vi "Unregister All.vi"() -> (3 "loggers":refnum<class "Logger.lvclass">[](array[class]))   [LabVIEW 2018, in "Logging.lvlib" / "Registry.lvlib"]
uses:
  Registry.lvlib
  Logger/Logger.lvclass
  Registry Actions.ctl
  Utilities/Utilities.lvlib
panel:
  # "Connector Pane"
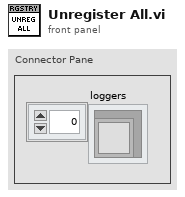
[diagram p1: front panel]
types:
  T1 = typedef "Logging.lvlib/Registry.lvlib/Registry Actions.ctl" = enum16{"Register", "Log", "Enable", "Enable All", "Disable", "Disable All", "List", "Unregister", "Unregister All"}
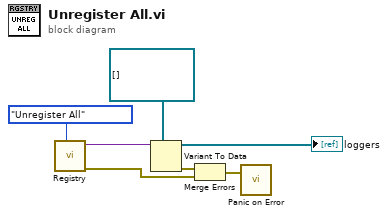
[diagram p0: block diagram]
diagram:
  n1 = call "Registry.vi"("action"=Registry_Actions."Unregister All") -> ("error out"=w2:errorcluster, "data out"=w6:variant)  [unwired: 9 in]
  n2 = Variant To Data(type=refnum<class "Logger.lvclass">[] [] ("Array"), Variant=w6) -> (data=→"loggers":refnum<class "Logger.lvclass">[], error out=w3:errorcluster)  [unwired: 1 in]
  n3 = Merge Errors(w3, w2) -> (w1:errorcluster)
  n4 = call "Panic on Error.vi"("error in (no error)"=w1) -> ()  [unwired: 3 in]
